vi "Day 18-Reduce.vi"(11 "Array in":i32[][](array[numeric])) -> (3 "Array out":i32[][](array[numeric]))   [LabVIEW 2021]
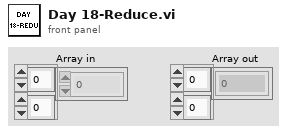
[diagram p1: front panel]
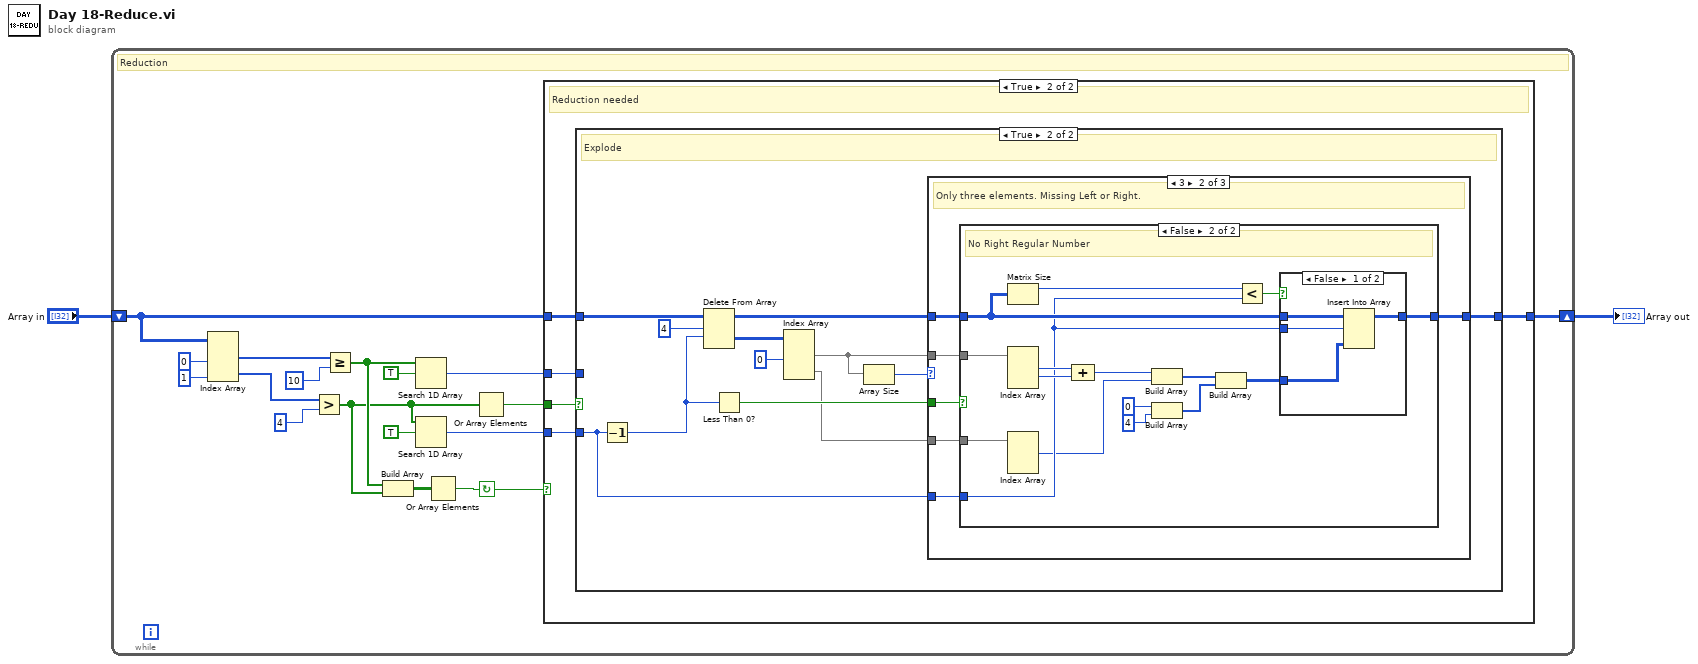
[diagram p0: block diagram]
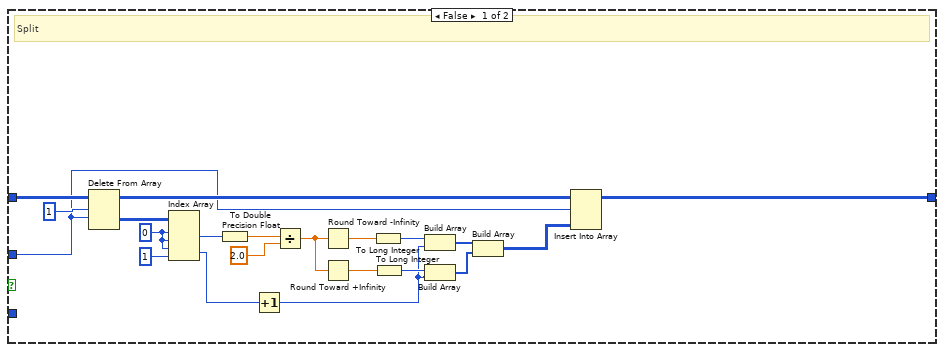
[diagram p3: hidden frame]
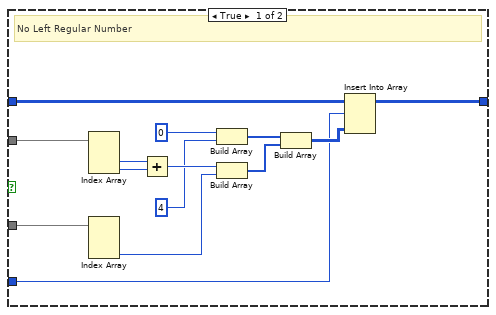
[diagram p5: hidden frame]
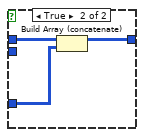
[diagram p6: hidden frame]
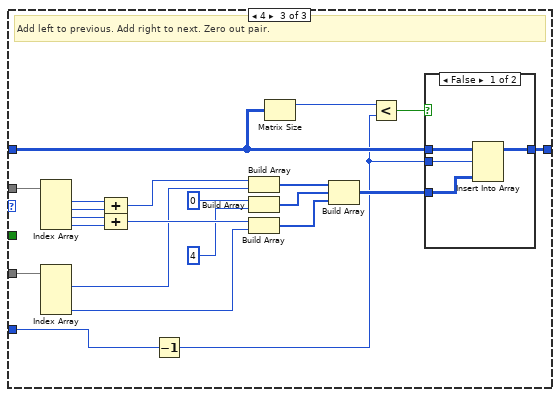
[diagram p7: hidden frame]
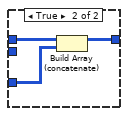
[diagram p8: hidden frame]
diagram:
  n1 = while {
    shift-right: [w15] -> w2
    shift-left: "Array in" -> [w9]
    stop <- w13 continue-if-true
    # "Reduction"
    n2 = Index Array(array=w9, index (col) #1=0 ("disabled index (col)"), index (col) #2=1 ("index (col)")) -> (element #1=w19:i32[], element #2=w18:i32[])  [unwired: 2 in]
    n3 = Greater?(x=w18, y=4) -> (0:w3:bool[])
    n4 = Greater Or Equal?(x=w19, y=10) -> (x >= y?=w6:bool[])
    n5 = Build Array(w6, w3) -> (w14:bool[][])
    n6 = Search 1D Array(1D array=w6, element=TRUE) -> (index of element=w5:i32)  [unwired: 1 in]
    n7 = Search 1D Array(1D array=w3, element=TRUE) -> (index of element=w4:i32)  [unwired: 1 in]
    n8 = Or Array Elements(Boolean array=w14) -> (logical OR=w13:bool)
    n9 = Or Array Elements(Boolean array=w3) -> (logical OR=w8:bool)
    n10 = case shown="True" w13 {
      tunnel: w9 -> [w20 w25]
      tunnel: [w20 w23] -> w15
      tunnel: w5 -> [_ w24]
      tunnel: w4 -> [_ w22]
      tunnel: w8 -> [_ w21]
      frame False {
        # "Reduction Complete"
      }
      frame True {
        # "Reduction needed"
        n11 = case shown="True" w21 {
          tunnel: w25 -> [w46 w47]
          tunnel: w24 -> [w29 _]
          tunnel: [w27 w49] -> w23
          tunnel: w22 -> [_ w50]
          frame False {
            w43 = 0 ("index (row)")
            # "Split"
            n12 = Delete From Array(array=w46, length=1, index (row)=w29) -> (deleted portion=w44:i32[][], array with subset deleted=w30:i32[][])  [unwired: 1 in]
            n13 = Index Array(array=w44, index (row) #1=w43, index (col) #1=w43, index (row) #2=w43, index (col) #2=1 ("disabled index (col)")) -> (element #1=w40:i32, element #2=w38:i32)
            n14 = To Double Precision Float(number=w40) -> (double precision float=w26:dbl)
            n15 = Increment(x=w38) -> (x+1=w33:i32)
            n16 = Divide(x=w26, y=2.0) -> (x/y=w39:dbl)
            n17 = Round Toward -Infinity(1:w39) -> (0:w37:dbl)
            n18 = Round Toward +Infinity(x=w39) -> (ceil(x): smallest int >= x=w35:dbl)
            n19 = To Long Integer(number=w37) -> (32bit integer=w36:i32)
            n20 = To Long Integer(number=w35) -> (32bit integer=w34:i32)
            n21 = Build Array(w36, w33) -> (w32:i32[])
            n22 = Build Array(w34, w33) -> (w31:i32[])
            n23 = Build Array(w32, w31) -> (w28:i32[][])
            n24 = Insert Into Array(array=w30, index (row)=w29, new element=w28) -> (w27:i32[][])  [unwired: 1 in]
          }
          frame True {
            # "Explode"
            n25 = Decrement(x=w50) -> (x-1=w55:i32)
            n26 = Delete From Array(array=w47, length=4, index (row)=w55) -> (deleted portion=w57:i32[][], array with subset deleted=w52:i32[][])  [unwired: 1 in]
            n27 = Less Than 0?(x=w55) -> (x < 0?=w54:bool)
            n28 = Index Array(array=w57, index (col) #1=0 ("disabled index (col)")) -> (element #1=w53:i32[], element #2=w48:i32[])  [unwired: 3 in]
            n29 = Array Size(array=w53) -> (size(s)=w51:i32)
            n30 = case shown="3" w51 {
              tunnel: w54 -> [_ w65 _]
              tunnel: w53 -> [_ w64 w124]
              tunnel: w52 -> [w59 w63 w107]
              tunnel: w50 -> [_ w62 w113]
              tunnel: [w59 w61 w115] -> w49
              tunnel: w48 -> [_ w60 w112]
              frame Default {
              }
              frame 3 {
                # "Only three elements. Missing Left or Right."
                n31 = case shown="False" w65 {
                  tunnel: w64 -> [w79 w95]
                  tunnel: w63 -> [w72 w85]
                  tunnel: w62 -> [w69 w83]
                  tunnel: [w71 w92] -> w61
                  tunnel: w60 -> [w68 w90]
                  frame True {
                    # "No Left Regular Number"
                    n32 = Index Array(array=w79) -> (element #2=w78:i32, element #3=w77:i32)  [unwired: 3 in, 1 out]
                    n33 = Index Array(array=w68) -> (element #3=w67:i32)  [unwired: 3 in, 2 out]
                    n34 = Add(x=w78, y=w77) -> (x+y=w75:i32)
                    n35 = Build Array(0 ("disabled index (col)"), 4 ("length")) -> (w74:i32[])
                    n36 = Build Array(w75, w67) -> (w73:i32[])
                    n37 = Build Array(w74, w73) -> (w70:i32[][])
                    n38 = Insert Into Array(array=w72, index (row)=w69, new element=w70) -> (w71:i32[][])  [unwired: 1 in]
                  }
                  frame False {
                    # "No Right Regular Number"
                    n39 = Matrix Size(0:w85) -> (1:w84:i32)  [unwired: 1 out]
                    n40 = Index Array(array=w95) -> (element #1=w89:i32, element #2=w88:i32)  [unwired: 3 in, 1 out]
                    n41 = Index Array(array=w90) -> (element #1=w81:i32)  [unwired: 3 in, 2 out]
                    n42 = Compound Arithmetic op=ADD(w89, w88) -> (w87:i32)
                    n43 = Build Array(w87, w81) -> (w94:i32[])
                    n44 = Build Array(0 ("disabled index (col)"), 4 ("length")) -> (w93:i32[])
                    n45 = Build Array(w94, w93) -> (w91:i32[][])
                    n46 = Less?(x=w84, y=w83) -> (x < y?=w82:bool)
                    n47 = case shown="False" w82 {
                      tunnel: w85 -> [w99 w102]
                      tunnel: [w98 w101] -> w92
                      tunnel: w91 -> [w97 w100]
                      tunnel: w83 -> [w96 _]
                      frame False {
                        n48 = Insert Into Array(array=w99, index (row)=w96, new element=w97) -> (w98:i32[][])  [unwired: 1 in]
                      }
                      frame True {
                        n49 = Build Array (concatenate)(w102, w100) -> (w101:i32[][])
                      }
                    }
                  }
                }
              }
              frame 4 {
                # "Add left to previous. Add right to next. Zero out pair."
                n50 = Index Array(array=w124) -> (element #1=w123:i32, element #2=w122:i32, element #3=w120:i32, element #4=w119:i32)  [unwired: 4 in]
                n51 = Index Array(array=w112) -> (element #1=w110:i32, element #4=w108:i32)  [unwired: 4 in, 2 out]
                n52 = Compound Arithmetic op=ADD(w123, w122) -> (w121:i32)
                n53 = Compound Arithmetic op=ADD(w120, w119) -> (w118:i32)
                n54 = Decrement(x=w113) -> (x-1=w105:i32)
                n55 = Build Array(w121, w110) -> (w116:i32[])
                n56 = Build Array(0 ("disabled index (col)"), 4 ("length")) -> (w109:i32[])
                n57 = Build Array(w118, w108) -> (w114:i32[])
                n58 = Matrix Size(0:w107) -> (1:w106:i32)  [unwired: 1 out]
                n59 = Build Array(w116, w109, w114) -> (w117:i32[][])
                n60 = Less?(x=w106, y=w105) -> (x < y?=w104:bool)
                n61 = case shown="False" w104 {
                  tunnel: w117 -> [w128 w129]
                  tunnel: [w127 w130] -> w115
                  tunnel: w107 -> [w126 w131]
                  tunnel: w105 -> [w125 _]
                  frame False {
                    n62 = Insert Into Array(array=w126, index (row)=w125, new element=w128) -> (w127:i32[][])  [unwired: 1 in]
                  }
                  frame True {
                    n63 = Build Array (concatenate)(w131, w129) -> (w130:i32[][])
                  }
                }
              }
            }
          }
        }
      }
    }
  }
  "Array out" <- w2
